vi "Get LibVLC path.vi"(0 "VLC Variables In":T1, 11 "error in (no error)":errorcluster) -> (4 "VLC Variables Out":T1, 15 "error out":errorcluster)   [LabVIEW 2012]
uses:
  Controls-Webcam/VLC Var.ctl
  <vilib>/registry/registry.llb/Registry RtKey.ctl
  <vilib>/registry/registry.llb/Registry SAM.ctl
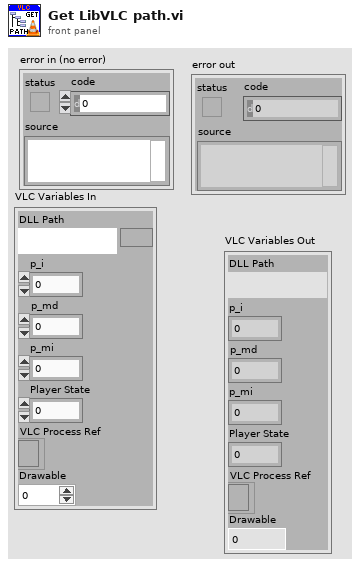
[diagram p1: front panel]
types:
  T1 = typedef "VLC Var.ctl" = cluster{"DLL Path":path, "p_i":i32, "p_md":i32, "p_mi":i32, "Player State":i32, "VLC Process Ref":refnum<k24>, "Drawable":i32}
  T2 = typedef "Registry SAM.ctl" = enum32{"KEY_QUERY_VALUE", "KEY_SET_VALUE", "KEY_CREATE_SUB_KEY", "KEY_ENUMERATE_SUB_KEYS", "KEY_NOTIFY", "KEY_CREATE_LINK", "KEY_READ", "KEY_WRITE", "KEY_ALL_ACCESS", "KEY_READ | KEY_WRITE"}
  T3 = typedef "Registry RtKey.ctl" = enum32{"HKEY_CLASSES_ROOT", "HKEY_CURRENT_USER", "HKEY_LOCAL_MACHINE", "HKEY_USERS", "HKEY_PERFORMANCE_DATA", "HKEY_CURRENT_CONFIG", "HKEY_DYN_DATA"}
  T4 = typedef "Registry refnum.ctl" = refnum<k1>
  T5 = cluster{"numValues":i32, "maxValueNameLen":i32, "maxValueDataLen":i32}
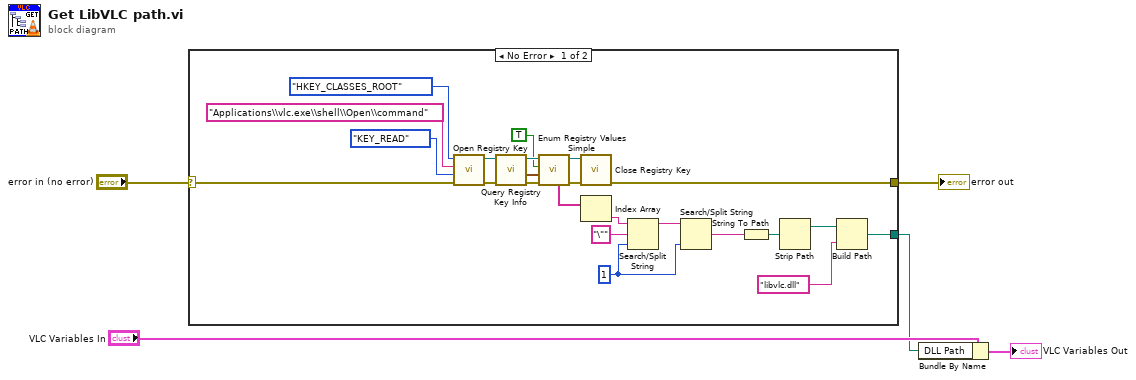
[diagram p0: block diagram]
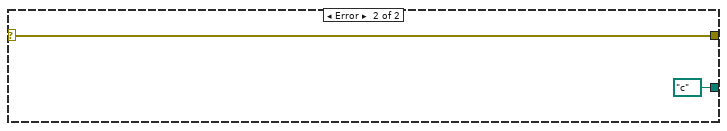
[diagram p2: hidden frame]
diagram:
  n1 = case shown="No Error" "error in (no error)" {
    selector: "error in (no error)" -> [w8 w30]
    tunnel: [w7 w30] -> w4
    tunnel: [w6 path "c:/" ("appended path")] -> w2
    frame No Error {
      w14 = 1 ("offset (0)")
      n2 = call <vilib>:"Open Registry Key.vi"("error in (no error)"=w8, "security access mask (KEY_READ | KEY_WRITE)"=Registry_SAM."KEY_READ", "subkey"="Applications\\vlc.exe\\shell\\Open\\command", "root key (HKEY_LOCAL_MACHINE)"=Registry_RtKey."HKEY_CLASSES_ROOT") -> ("error out"=w24:errorcluster, "refnum out"=w25:T4)  [unwired: 6 in]
      n3 = call <vilib>:"Query Registry Key Info.vi"("error in (no error)"=w24, "refnum"=w25) -> ("error out"=w22:errorcluster, "value info"=w21:T5, "refnum out"=w23:T4)  [unwired: 5 in, 2 out]
      n4 = call <vilib>:"Enum Registry Values Simple.vi"("error in (no error)"=w22, "value info"=w21, "retrieve data? (F)"=TRUE, "refnum"=w23) -> ("error out"=w18:errorcluster, "refnum out"=w19:T4, "String/Binary data"=w17:string[])  [unwired: 2 in, 3 out]
      n5 = call <vilib>:"Close Registry Key.vi"("error in (no error)"=w18, "refnum"=w19) -> ("error out"=w7:errorcluster)  [unwired: 5 in]
      n6 = Index Array(array=w17) -> (element=w16:string)  [unwired: 1 in]
      n7 = Search/Split String(string=w16, search string/char (-)="\"", offset (0)=w14) -> (substring before match=w15:string)  [unwired: 2 out]
      n8 = Search/Split String(string=w15, offset (0)=w14) -> (match + rest of string=w9:string)  [unwired: 1 in, 2 out]
      n9 = String To Path(string=w9) -> (path=w11:path)
      n10 = Strip Path(path=w11) -> (stripped path=w10:path)  [unwired: 1 out]
      n11 = Build Path(base path=w10, name or relative path="libvlc.dll") -> (appended path=w6:path)
    }
    frame Error {
    }
  }
  "error out" <- w4
  n12 = Bundle By Name(cluster="VLC Variables In", "DLL Path"=w2) -> (→"VLC Variables Out":T1)
